vi "test_MultisitePinMapARegistered_ReserveSessionTwice_SecondReserveFails.vi"() -> (6 "pass":bool, 8 "result":string, 15 "error out":errorcluster)   [LabVIEW 2020]
uses:
  Runtime/MeasurementLink Pin Map Client/RPC Messages/ni_measurementlink_pinmap_v1_CreatePinMapFromXmlRequest.ctl
  Runtime/MeasurementLink Session Management Client/RPC Messages/ni_measurementlink_sessionmanagement_v1_ReserveSessionsRequest.ctl
  Runtime/MeasurementLink Session Management Client/RPC Messages/ni_measurementlink_PinMapContext.ctl
  Runtime/MeasurementLink Session Management Client/RPC Messages/ni_measurementlink_sessionmanagement_v1_ReserveAllRegisteredSessionsResponse.ctl
  Runtime/MeasurementLink Session Management Client/RPC Messages/ni_measurementlink_sessionmanagement_v1_SessionInformation.ctl
  Runtime/MeasurementLink Session Management Client/RPC Messages/nidevice_grpc_Session.ctl
  Runtime/MeasurementLink Session Management Client/RPC Messages/ni_measurementlink_sessionmanagement_v1_ChannelMapping.ctl
  Runtime/MeasurementLink Session Management Client/MeasurementLink Session Management Client.lvlib
  Runtime/MeasurementLink Pin Map Client/MeasurementLink Pin Map Client.lvlib
panel:
  # "Test assumes discovery service, pin map service, and session management service have already been started."
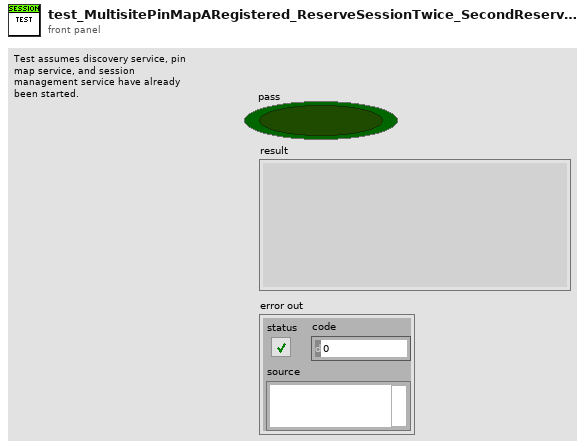
[diagram p1: front panel]
types:
  T1 = typedef "MeasurementLink Session Management Client.lvlib/ni_measurementlink_sessionmanagement_v1_ReserveAllRegisteredSessionsResponse.ctl" = cluster{"sessions":T2[]}
  T2 = typedef "MeasurementLink Session Management Client.lvlib/ni_measurementlink_sessionmanagement_v1_SessionInformation.ctl" = cluster{"session":T3, "resource_name":string, "channel_list":string, "instrument_type_id":string, "session_exists":bool, "channel_mappings":T4[]}
  T3 = typedef "MeasurementLink Session Management Client.lvlib/nidevice_grpc_Session.ctl" = cluster{"name":string}
  T4 = typedef "MeasurementLink Session Management Client.lvlib/ni_measurementlink_sessionmanagement_v1_ChannelMapping.ctl" = cluster{"pin_or_relay_name":string, "site":i32, "channel":string, "multiplexer_resource_name":string, "multiplexer_route":string}
  T5 = typedef "MeasurementLink Session Management Client.lvlib/ni_measurementlink_sessionmanagement_v1_ReserveSessionsRequest.ctl" = cluster{"pin_map_context":T6, "pin_or_relay_names":string[], "instrument_type_id":string, "timeout_in_milliseconds":i32}
  T6 = typedef "MeasurementLink Session Management Client.lvlib/ni_measurementlink_PinMapContext.ctl" = cluster{"pin_map_id":string, "sites":i32[]}
  T7 = typedef "MeasurementLink Pin Map Client.lvlib/ni_measurementlink_pinmap_v1_CreatePinMapFromXmlRequest.ctl" = cluster{"pin_map_id":string, "pin_map_xml":string}
  T8 = typedef "grpc-lvsupport-release.lvlib/grpcId.ctl" = u64
  T9 = typedef "MeasurementLink Session Management Client.lvlib/ni_measurementlink_sessionmanagement_v1_ReserveSessionsResponse.ctl" = cluster{"sessions":T2[], "multiplexer_sessions":T10[]}
  T10 = typedef "MeasurementLink Session Management Client.lvlib/ni_measurementlink_sessionmanagement_v1_MultiplexerSessionInformation.ctl" = cluster{"session":T3, "resource_name":string, "multiplexer_type_id":string, "session_exists":bool}
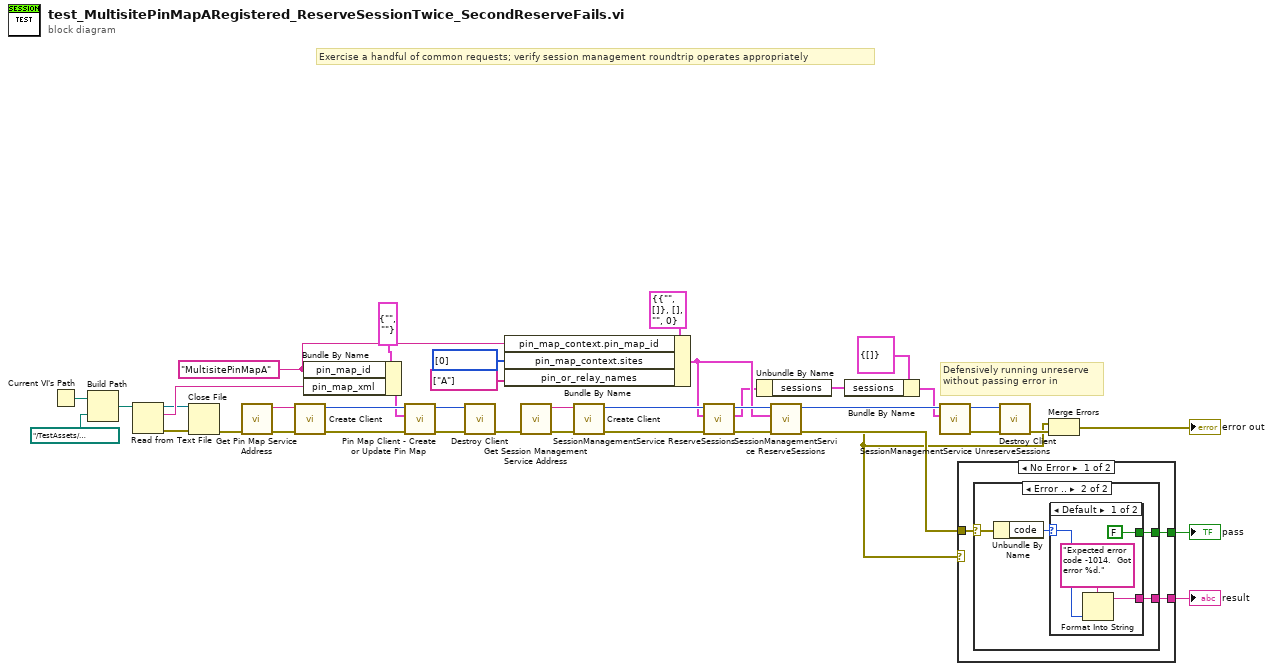
[diagram p0: block diagram]
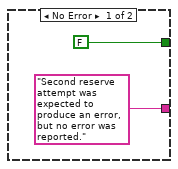
[diagram p2: hidden frame]
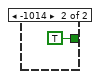
[diagram p3: hidden frame]
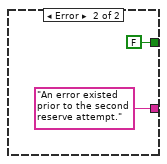
[diagram p4: hidden frame]
diagram:
  w17 = "MultisitePinMapA" ("pin_map_id")
  # "Defensively running unreserve without passing error in"
  # "Exercise a handful of common requests; verify session management roundtrip operates appropriately"
  n1 = Current VI's Path() -> (path=w34:path)
  n2 = Build Path(base path=w34, name or relative path=path "../TestAssets/MultisitePinMapA-3Instruments_3DutPins_2SystemPins_2Sites.pinmap") -> (appended path=w32:path)
  n3 = Read from Text File(file (use dialog)=w32) -> (refnum out=w28:refnum<file>, text=w30:string, error out=w29:errorcluster)  [unwired: 3 in, 1 out]
  n4 = Close File(refnum=w28, error in=w29) -> (error out=w25:errorcluster)  [unwired: 1 out]
  n5 = call "Get Pin Map Service Address.vi"("error in (no error)"=w25) -> ("error out"=w26:errorcluster, "address"=w27:string)  [unwired: 9 in]
  n6 = call "Create Client.vi"("error in"=w26, "address"=w27) -> ("error out"=w35:errorcluster, "gRPC ID Out"=w24:T8)  [unwired: 8 in]
  n7 = Bundle By Name(cluster=T7 {"pin_map_id"="", "pin_map_xml"=""} ("Request Data"), "pin_map_id"=w17, "pin_map_xml"=w30) -> (w23:T7)
  n8 = call "Pin Map Client - Create or Update Pin Map.vi"("error in (no error)"=w35, "Request Data"=w23, "gRPC ID Out"=w24) -> ("error out"=w22:errorcluster, "gRPC ID out"=w21:T8)  [unwired: 6 in, 1 out]
  n9 = call "Destroy Client.vi"("error in"=w22, "gRPC ID"=w21) -> ("error out"=w20:errorcluster)  [unwired: 9 in]
  n10 = Bundle By Name(cluster=T5 {"pin_map_context"={"pin_map_id"="", "sites"=[]}, "pin_or_relay_names"=[], "instrument_type_id"="", "timeout_in_milliseconds"=0} ("Request Data"), "pin_map_context.pin_map_id"=w17, "pin_map_context.sites"=i32[] [0], "pin_or_relay_names"=string[] ["A"]) -> (w11:T5)
  n11 = call "Get Session Management Service Address.vi"("error in (no error)"=w20) -> ("error out"=w39:errorcluster, "address"=w38:string)  [unwired: 9 in]
  n12 = call "Create Client.vi"("error in"=w39, "address"=w38) -> ("error out"=w37:errorcluster, "gRPC ID Out"=w36:T8)  [unwired: 8 in]
  n13 = call "SessionManagementService ReserveSessions.vi"("error in"=w37, "Request Data"=w11, "gRPC ID"=w36) -> ("error out"=w5:errorcluster, "Response Data"=w4:T9, "gRPC ID out"=w13:T8)  [unwired: 6 in]
  n14 = Unbundle By Name(w4) -> ("sessions"=w2:T2[])
  n15 = call "SessionManagementService ReserveSessions.vi"("error in"=w5, "Request Data"=w11, "gRPC ID"=w13) -> ("error out"=w8:errorcluster, "gRPC ID out"=w12:T8)  [unwired: 6 in, 1 out]
  n16 = Bundle By Name(cluster=T1 {"sessions"=[]} ("response data 2"), "sessions"=w2) -> (w1:T1)
  n17 = call "SessionManagementService UnreserveSessions.vi"("Request Data"=w1, "gRPC ID"=w12) -> ("error out"=w14:errorcluster, "gRPC ID out"=w19:T8)  [unwired: 7 in, 1 out]
  n18 = case shown="No Error" w5 {
    tunnel: [w42 FALSE] -> w10
    tunnel: [w41 "An error existed prior to the second reserve attempt." ("String")] -> w9
    tunnel: w8 -> [w40 _]
    frame No Error {
      n19 = case shown="Error .." w40 {
        selector: w40 -> [_ w48]
        tunnel: [FALSE w45] -> w42
        tunnel: ["Second reserve attempt was expected to produce an error, but no error was reported." ("String") w46] -> w41
        frame No Error {
        }
        frame Error {
          n20 = Unbundle By Name(w48) -> ("code"=w47:i32)
          n21 = case shown="Default" w47 {
            selector: w47 -> [w49 _]
            tunnel: [w51 _] -> w46
            tunnel: [FALSE TRUE] -> w45
            frame Default {
              n22 = Format Into String(format string="Expected error code -1014.  Got error %d." ("String"), w49) -> (resulting string=w51:string)  [unwired: 2 in, 1 out]
            }
            frame -1014 {
            }
          }
        }
      }
    }
    frame Error {
    }
  }
  "pass" <- w10
  "result" <- w9
  n23 = call "Destroy Client.vi"("error in"=w14, "gRPC ID"=w19) -> ("error out"=w7:errorcluster)  [unwired: 9 in]
  n24 = Merge Errors(w5, w7) -> (→"error out":errorcluster)
